vi "STM_CRC32.vi"(10 "crc (0xFFFFFFFF)":u32=4294967295 format="%.0x", 11 "buffer":u8[](array[numeric]) format="%.0x") -> (3 "crc":u32 format="%.0x")   [LabVIEW 2019]
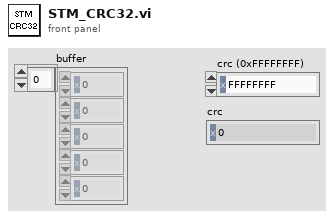
[diagram p1: front panel]
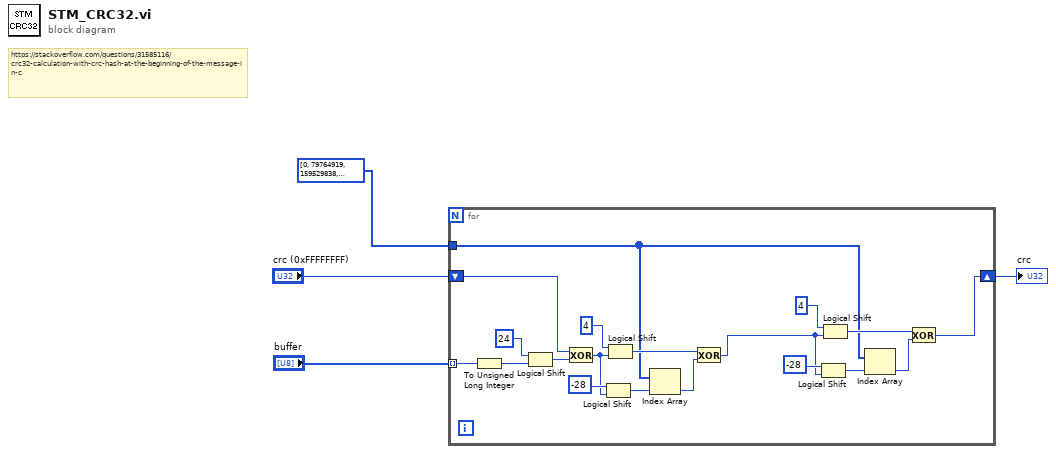
[diagram p0: block diagram]
diagram:
  # "https://stackoverflow.com/questions/31585116/crc32-calculation-with-crc-hash-at-the-beginning-of-the-message-in-c"
  n1 = for {
    tunnel: "buffer" -> [w23] mode=indexing
    shift-right: [w6] -> w2
    shift-left: "crc (0xFFFFFFFF)" -> [w19]
    tunnel: u32[] [0, 79764919, 159529838, 222504665, 319059676, 398814059, 445009330, 507990021, 638119352, 583659535, 797628118, 726387553, 890018660, 835552979, 1015980042, 944750013] -> [w5]
    n2 = To Unsigned Long Integer(number=w23) -> (unsigned 32bit integer=w22:u32)
    n3 = Logical Shift(y=i16 24, x=w22) -> (x << y=w20:u32)
    n4 = Exclusive Or(1:w20, 2:w19) -> (0:w15:u32)
    n5 = Logical Shift(y=i16 -28, x=w15) -> (x << y=w14:u32)
    n6 = Logical Shift(y=i16 4, x=w15) -> (x << y=w17:u32)
    n7 = Index Array(array=w5, index=w14) -> (element=w13:u32)
    n8 = Exclusive Or(1:w13, 2:w17) -> (0:w7:u32)
    n9 = Logical Shift(y=i16 -28, x=w7) -> (x << y=w9:u32)
    n10 = Logical Shift(y=i16 4, x=w7) -> (x << y=w11:u32)
    n11 = Index Array(array=w5, index=w9) -> (element=w8:u32)
    n12 = Exclusive Or(1:w8, 2:w11) -> (0:w6:u32)
  }
  "crc" <- w2
